vi "CalculateUnbalance.vi"(8 "error in (no error)":errorcluster, 11 "3-phase waveforms":waveform(dbl)[](array[waveform])) -> (0 "error out":errorcluster, 3 "unbalance [%]":dbl)   [LabVIEW 2017, in "McsaAnalysisFunctions.lvlib"]
uses:
  <vilib>/addons/InsightCM/Utilities/Analysis/MCSA/McsaAnalysisFunctions.lvlib
  <vilib>/addons/Electrical Power/Basic/NI_EP_Basic.lvlib
  <vilib>/addons/Electrical Power/Motor Monitoring/NI_EP_Motor Monitoring.lvlib
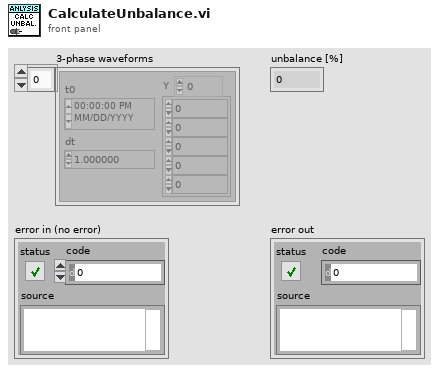
[diagram p1: front panel]
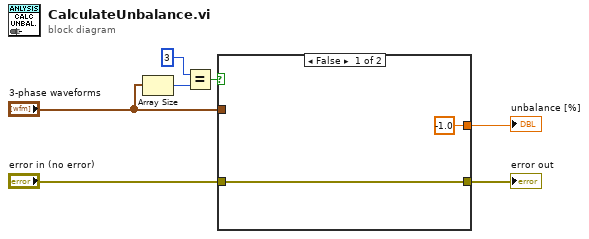
[diagram p0: block diagram]
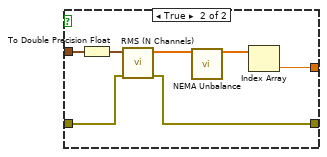
[diagram p2: hidden frame]
diagram:
  n1 = Array Size(array="3-phase waveforms") -> (size(s)=w3:i32)
  n2 = Equal?(x=3, y=w3) -> (x = y?=w4:bool)
  n3 = case shown="False" w4 {
    tunnel: [w8 w16] -> w7
    tunnel: "3-phase waveforms" -> [_ w12]
    tunnel: [-1.0 ("NEMA derating factor") w11] -> w6
    tunnel: "error in (no error)" -> [w8 w10]
    frame False {
    }
    frame True {
      n4 = To Double Precision Float(number=w12) -> (double precision float=w15:waveform(dbl)[])
      n5 = call <vilib>:"RMS (N Channels).vi"("error in (no error)"=w10, "waveforms"=w15) -> ("error out"=w16:errorcluster, "RMS values"=w13:dbl[])  [unwired: 8 in]
      n6 = call <vilib>:"NEMA Unbalance.vi"("voltage RMS values"=w13) -> ("unbalance [%]"=w14:dbl[])  [unwired: 12 in, 2 out]
      n7 = Index Array(array=w14) -> (element=w11:dbl)  [unwired: 1 in]
    }
  }
  "error out" <- w7
  "unbalance [%]" <- w6
